vi "Live window-Enable image.vi"(9 "Enable":bool, 11 "Which image display?":T1) -> ()   [LabVIEW 2020]
uses:
  Typedefs/Left-Right enum.ctl
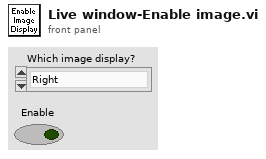
[diagram p1: front panel]
types:
  T1 = typedef "Left-Right enum.ctl" = enum16{"Right", "Left"}
  T2 = enum8{"Enabled", "Disabled", "Disabled and Grayed Out"}
  T3 = typedef "Image display ref.ctl" = refnum<vi>
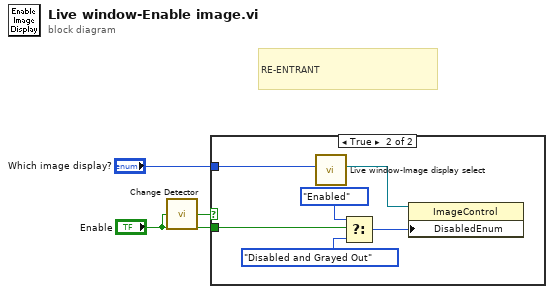
[diagram p0: block diagram]
diagram:
  # "RE-ENTRANT"
  n1 = call <userlib>:"Change Detector.vi"("Value"="Enable") -> ("Changed?"=w2:bool)
  n2 = case shown="True" w2 {
    tunnel: "Enable" -> [_ w9]
    tunnel: "Which image display?" -> [_ w4]
    frame False {
    }
    frame True {
      n3 = call "Live window-Image display select.vi"("Which image display?"=w4) -> ("Image display ref"=w5:T3)  [unwired: 10 in]
      n4 = Select(t=T2."Enabled" ("Disabled"), s=w9, f=T2."Disabled and Grayed Out" ("Disabled")) -> (s? t:f=w6:T2)
      n5 = property on="Property Node" class="ImageControl"(reference=w5, "DisabledEnum"=w6) -> ()  [unwired: 1 in, 2 out]
    }
  }
